vi "SpectrumAWG.vi"() -> ()   [LabVIEW 2014]
uses:
  Chart.ctl
  Wave.ctl
  spcm_library/spcm_gui_m4i.llb/element_ao_trigger.ctl
  spcm_library/spcm_gui_m4i.llb/element_clock.ctl
  spcm_library/spcm_gui_m4i.llb/element_ao_channel.ctl
  spcm_library/spcm_gui_m4i.llb/element_mode_out.ctl
panel:
  in  "Back":bool
  out "Wave Backup":T1 {"Phase (Pi)" min=-1.0 max=1.0 step=0.1 format="%.2f"; "Gap (us)" format="%.2f"; "Amplitude" format="%.2f"; "Duration (us)" format="%.2f"; "Frequency (MHz)" format="%.4f"}
  out "Card":cluster{"Card Handle":u64, "Error Code":u32}
  in  "Single":bool=TRUE
  in  "Formula":string="a*sin(w*t)" caption="data file"
  in  "Gap (us)":dbl=0.001 format="%.2f"
  in  "Phase (Pi)":dbl min=-1.0 max=1.0 step=0.1 format="%.2f"
  in  "Amplitude":dbl=1.0 format="%.2f"
  in  "Duration (us)":dbl=1.0 format="%.3f"
  in  "Frequency (MHz)":dbl=200.0 format="%.4f"
  in  "Output Channel":T2={"Enable"=TRUE, "Output Mode"=0, "Gain"=300, "Offset"=0, "Filter"=0} {"Output Mode" items=["Single", "Double", "Differential"]}
  in  "Mode":T3(ring)=enum."Single Restart"
  out "Status":string
  in  "Clock Settings":T4={"Clock Mode"=1, "Sampling Rate (MHz)"=1000.0, "Reference Clock (MHz)"=10.0, "Clock Output"=FALSE} {"Clock Mode" items=["Internal Clock Quartz", "External Clock (Reference Clock)", "Quartz 2 with PLL (Optional)"]; "Reference Clock (MHz)" min=10.0 max=125000.0; "Sampling Rate (MHz)" min=1.0 max=200000.0}
  in  "Trigger Settings":T5={"Trigger Source"=1, "Main Ext. Trigger"=2, "Level 0 Ext"=0, "Level 1 Ext"=0, "AC Coupling"=0, "Ext Trig Term"=FALSE, "Secondary Ext. Trigger"=0, "Level 0 Ext1"=0, "Trigger Delay (Samples)"=0} {"Secondary Ext. Trigger" items=["None", "Pos. Edge", "Neg. Edge", "Any Edge", "High Level", "Low Level"]; "AC Coupling" items=["DC Coupling", "AC Coupling"]; "Main Ext. Trigger" items=["None", "Pos. Edge", "Neg. Edge", "Any Edge", "Pos. Rearm", "Neg. Rearm", "Enter Window", "Leave Window", "High Level", "Low Level", "In Win", "Out Win", ""]; "Trigger Source" items=["Software Trigger", "Main External Trigger", "Secondary External Trigger"]; "Trigger Delay (Samples)" max=65535 step=1}
  in  "Sync":bool
  in  "Row":u16(ring) items=["0"]
  in  "Action":bool
  in  "Save":bool
  in  "SegmentPositions":i32[](array[numeric])
  in  "Wave File":path
  in  "Quit":bool
  in  "Steps":T6(array[cluster]) {"End" max=1 step=1}
  in  "Segment":u16(ring) items=["0"]
  out "Wave":T1 {"Phase (Pi)" min=-1.0 max=1.0 step=0.1 format="%.2f"; "Gap (us)" format="%.2f"; "Amplitude" format="%.2f"; "Duration (us)" format="%.3f"; "Frequency (MHz)" format="%.4f"}
  in  "Wave String":string="Frequency (MHz),Duration (us),Amplitude,Phase (Pi),Gap (us),Formula\n39,0,0.5,0,0,\n41,0,0.5,0,0,\n0,10,1,0,0,[0 1]"
  out "Plot":T7
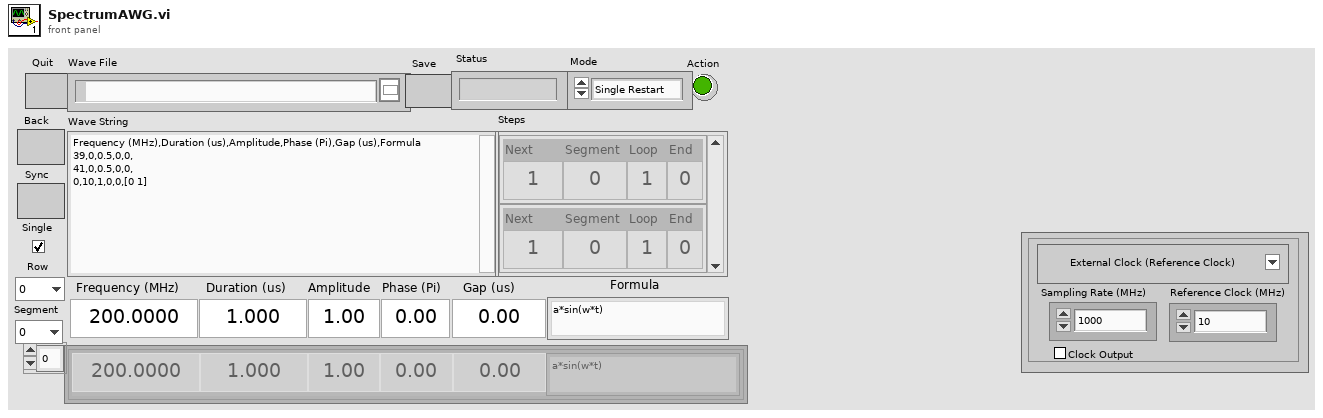
[diagram p1: front panel]
types:
  T1 = typedef "Wave.ctl" = cluster{"Frequency (MHz)":dbl, "Duration (us)":dbl, "Amplitude":dbl, "Phase (Pi)":dbl, "Gap (us)":dbl, "Formula":string}[]
  T2 = typedef "element_ao_channel.ctl" = cluster{"Enable":bool, "Output Mode":u16, "Gain":i32, "Offset":i32, "Filter":i32}
  T3 = enum16{"Singleshot", "Continuous", "Single Restart", "Multiple Replay", "Gated Replay"}
  T4 = typedef "element_clock.ctl" = cluster{"Clock Mode":u16, "Sampling Rate (MHz)":dbl, "Reference Clock (MHz)":dbl, "Clock Output":bool}
  T5 = typedef "element_ao_trigger.ctl" = cluster{"Trigger Source":u16, "Main Ext. Trigger":u16, "Level 0 Ext":i32, "Level 1 Ext":i32, "AC Coupling":u16, "Ext Trig Term":bool, "Secondary Ext. Trigger":u16, "Level 0 Ext1":i32, "Trigger Delay (Samples)":u32}
  T6 = cluster{"Next":u32, "Segment":u32, "Loop":u32, "End":u32}[]
  T7 = typedef "Chart.ctl" = waveform(dbl)
  T8 = cluster{"Index":u32, "IP Address":string, "Device":u16}
  T9 = cluster{"Next":u32, "Segment":u32, "Loop":u32, "End":u32}
  T10 = cluster{"Frequency (MHz)":dbl, "Duration (us)":dbl, "Amplitude":dbl, "Phase (Pi)":dbl, "Gap (us)":dbl, "Formula":string}
  T11 = typedef "element_mode_out.ctl" = cluster{"Mode":u16, "Mem":u32, "Seg":u32, "Loop":u32}
  T12 = cluster{"Number of segments":u32, "Start segment":u32}
  T13 = cluster{"Step":i32, "Next Step":i32, "Segment":i32, "Loops":i32, "End condition":u16}
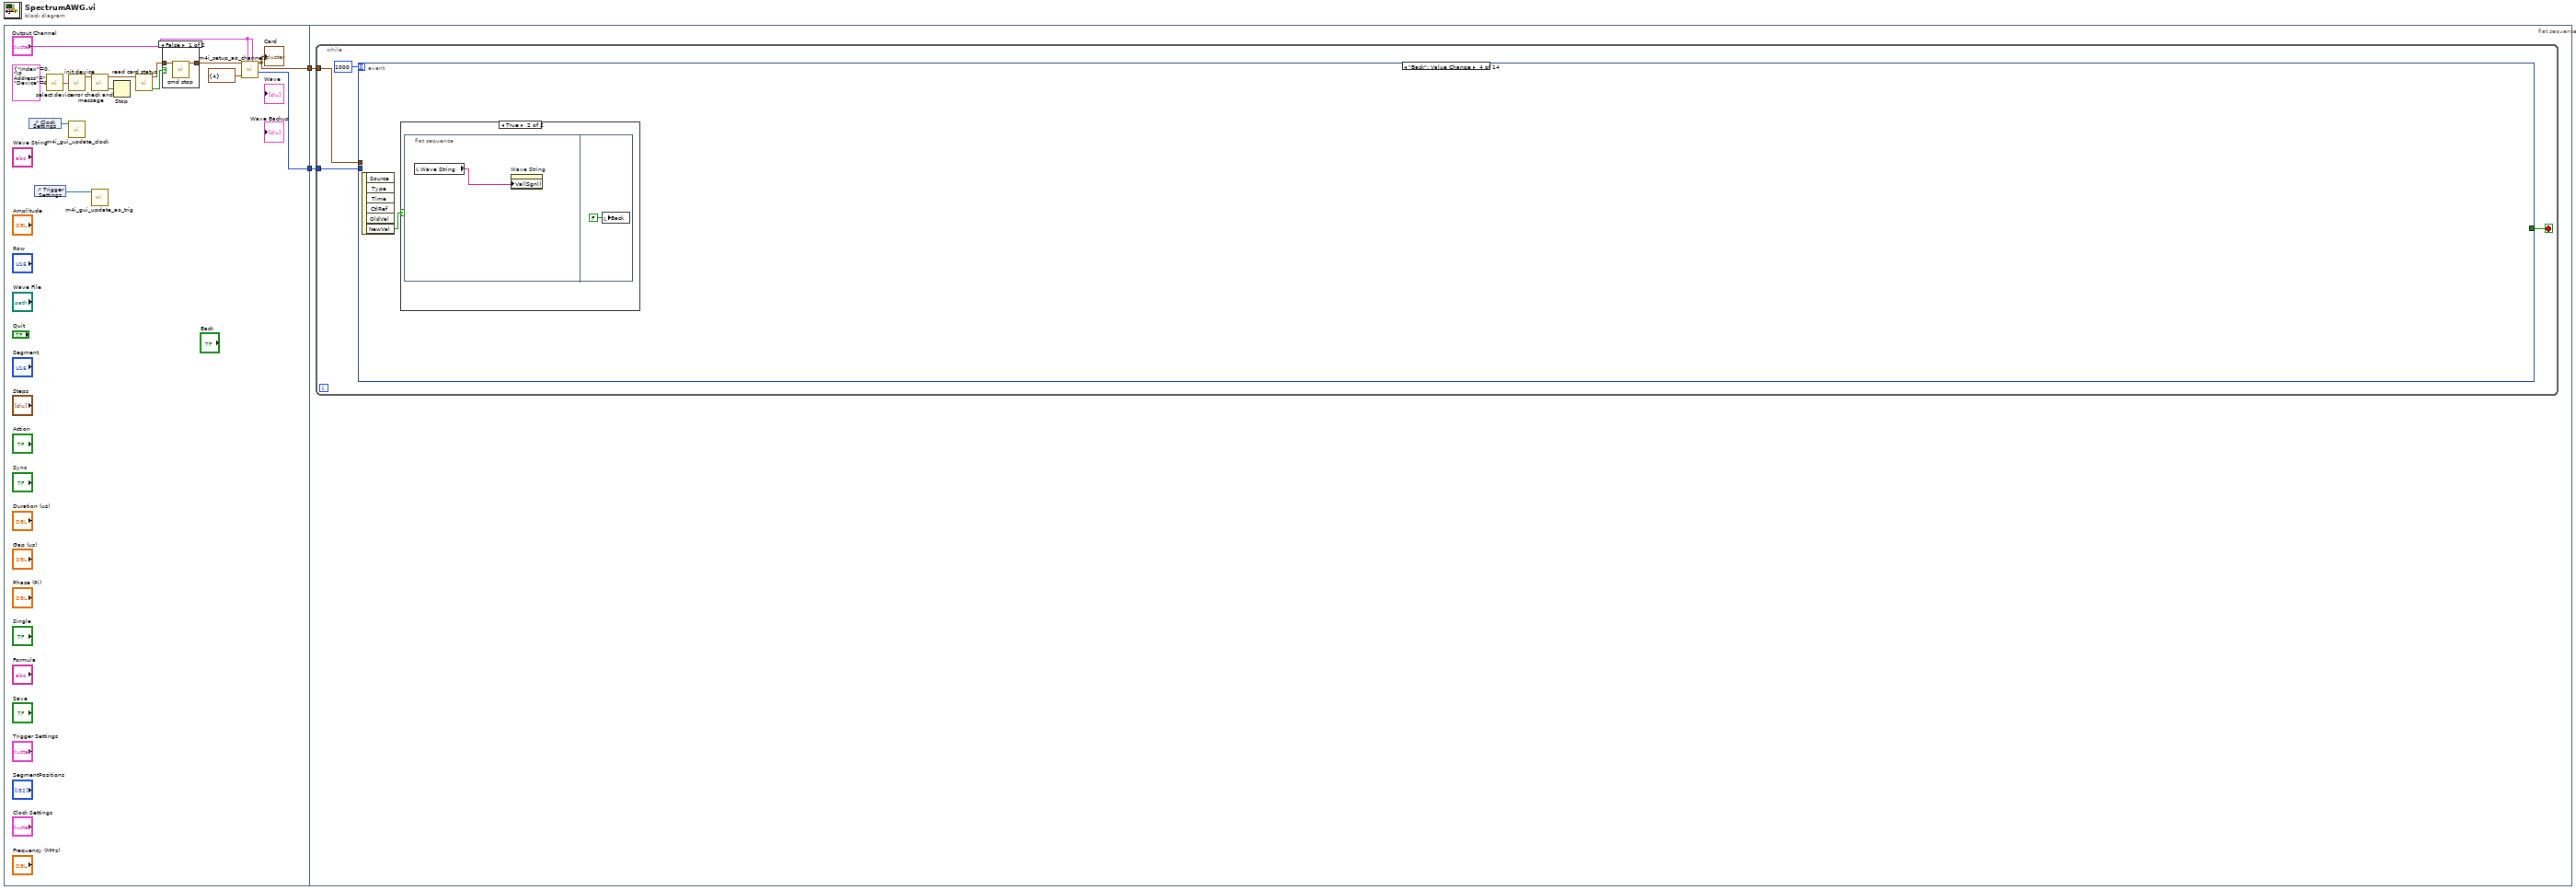
[diagram p0: block diagram]
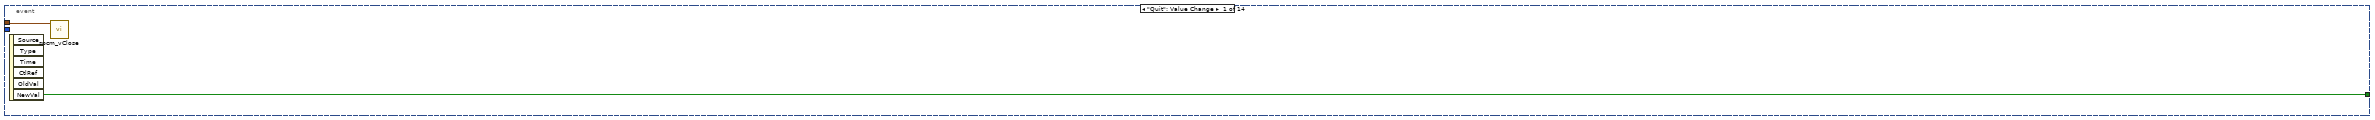
[diagram p3: hidden frame]
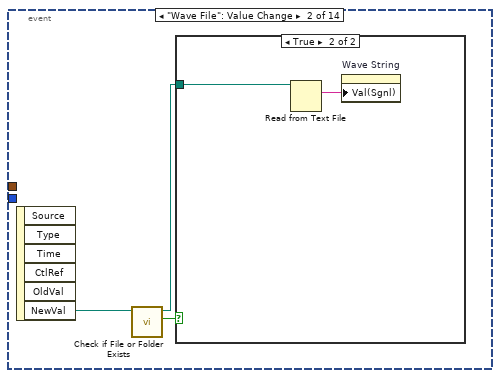
[diagram p4: hidden frame]
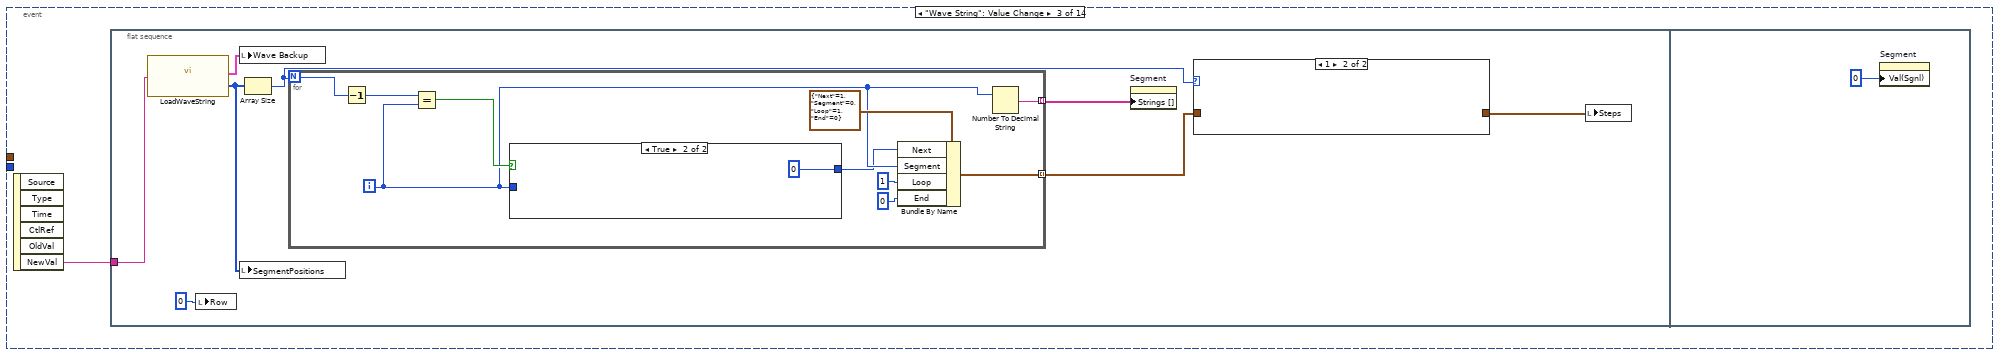
[diagram p6: hidden frame]
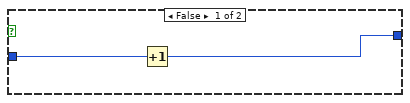
[diagram p8: hidden frame]
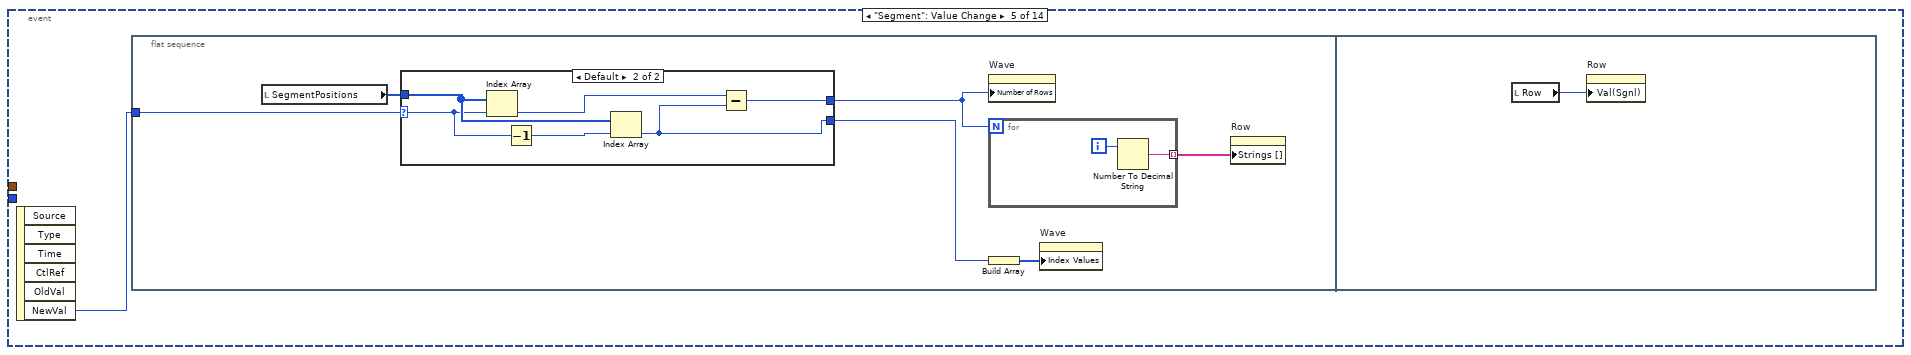
[diagram p10: hidden frame]
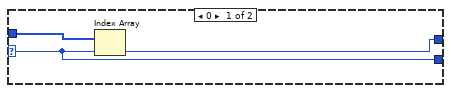
[diagram p11: hidden frame]
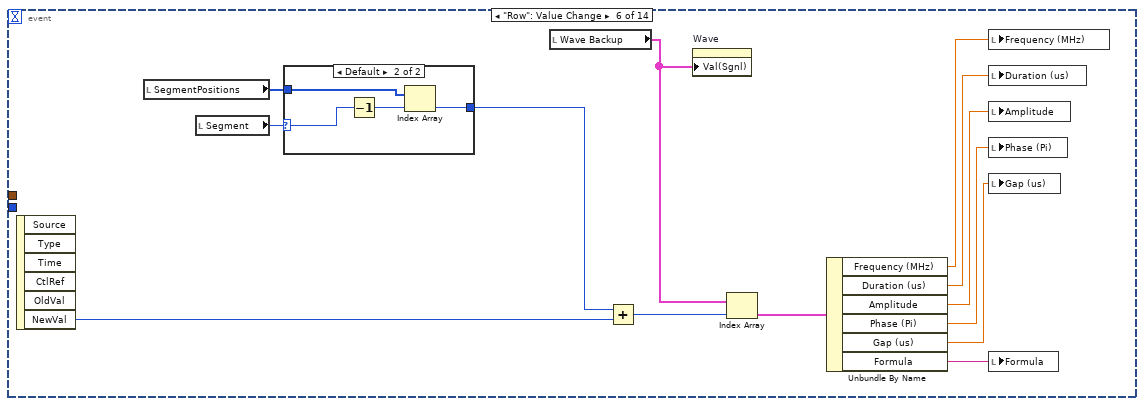
[diagram p12: hidden frame]
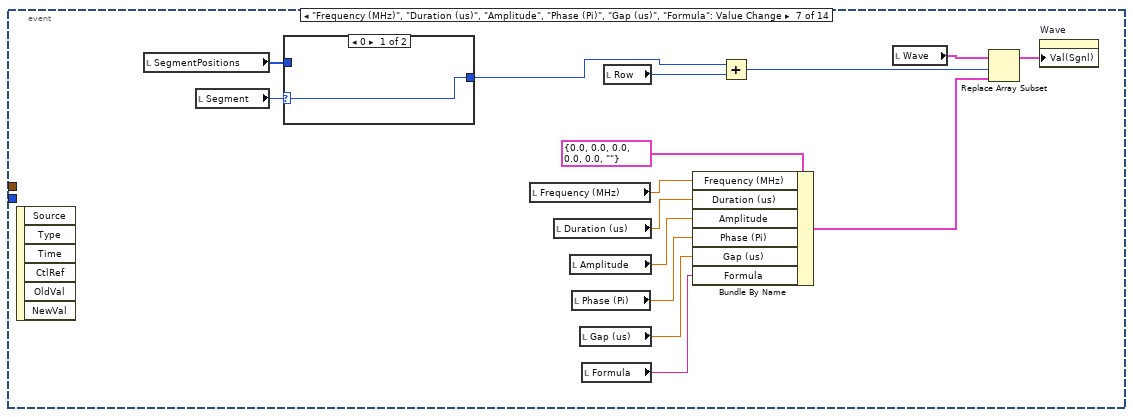
[diagram p14: hidden frame]
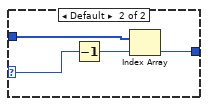
[diagram p15: hidden frame]
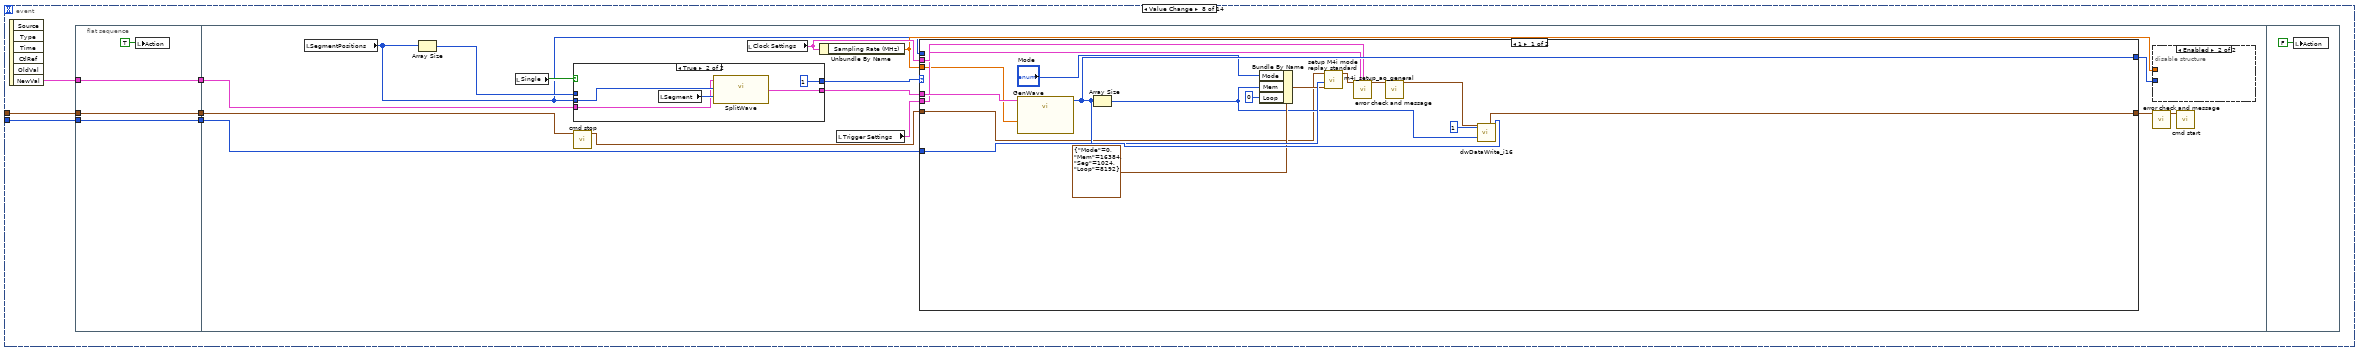
[diagram p16: hidden frame]
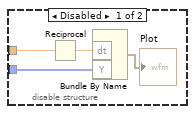
[diagram p18: hidden frame]
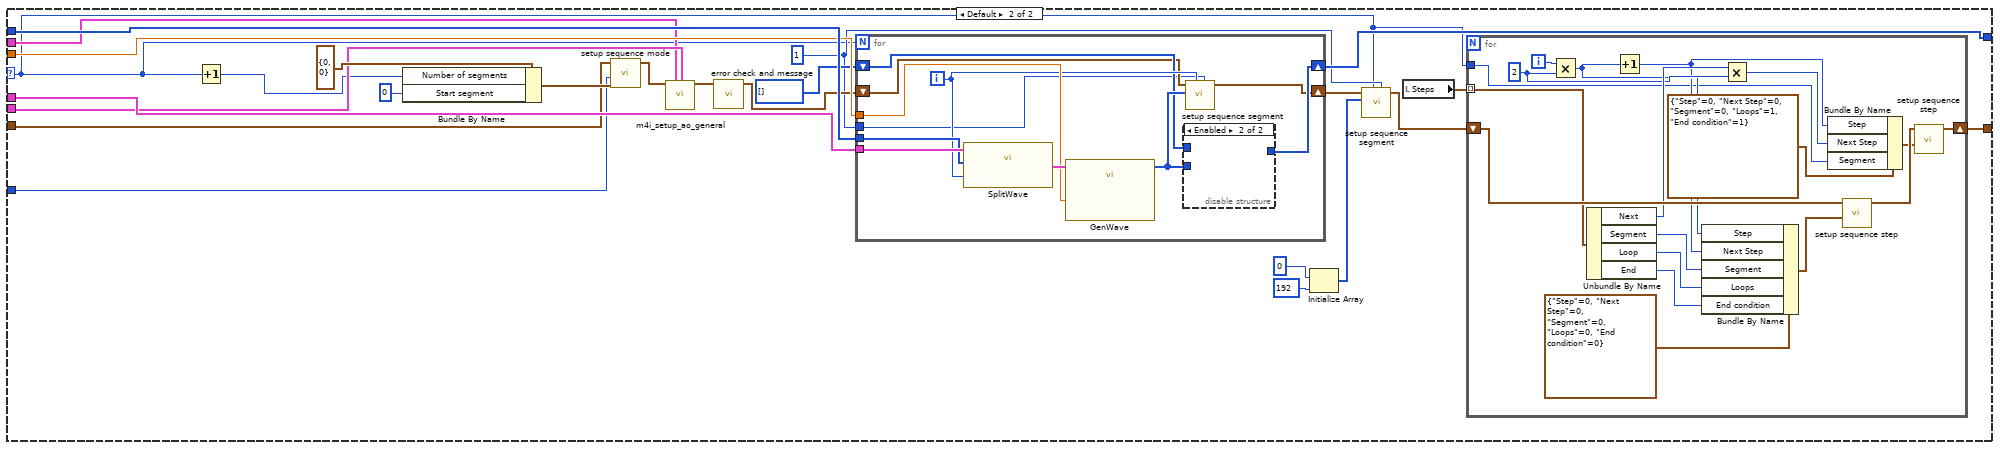
[diagram p19: hidden frame]
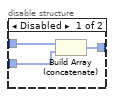
[diagram p20: hidden frame]
diagram:
  n1 = flat-sequence {
    tunnel: [w6] -> w2
    tunnel: [w3] -> w1
    tunnel: w2 -> [w21]
    tunnel: w1 -> [w20]
    frame #0 {
      n2 = control-ref of="Clock Settings"() -> (w7:refnum<vi>)
      n3 = control-ref of="Trigger Settings"() -> (w8:refnum<vi>)
      n4 = call "select device.vi"("Device"=T8 {"Index"=0, "IP Address"="", "Device"=0}) -> ("device string"=w16:string)  [unwired: 4 in]
      n5 = call "init device.vi"("Device String"=w16) -> ("Card Info Out"=w15:cluster{"Card Handle":u64, "Error Code":u32})  [unwired: 4 in, 1 out]
      n6 = call "m4i_gui_update_clock.vi"("Cluster Reference"=w7) -> ()  [unwired: 11 in]
      n7 = call "error check and message.vi"("Card Info In"=w15) -> ("Error occurred"=w14:bool, "Card Info Out"=w10:cluster{"Card Handle":u64, "Error Code":u32})  [unwired: 4 in, 1 out]
      n8 = call "m4i_gui_update_ao_trig.vi"("Cluster Referenz"=w8) -> ()  [unwired: 11 in]
      n9 = Stop(stop? (T)=w14) -> ()
      n10 = call "read card status.vi"("Card Info In"=w10) -> ("Card ready"=w11:bool, "Card Info Out"=w12:cluster{"Card Handle":u64, "Error Code":u32})  [unwired: 3 in, 2 out]
      n11 = case shown="False" w11 {
        tunnel: w12 -> [w18 w19]
        tunnel: [w17 w19] -> w9
        frame False {
          n12 = call "cmd stop.vi"("Card Info In"=w18) -> ("Card Info Out"=w17:cluster{"Card Handle":u64, "Error Code":u32})  [unwired: 6 in]
        }
        frame True {
        }
      }
      n13 = call "m4i_setup_ao_channels.vi"("Output Channel 1"="Output Channel", "Output Channel 0"="Output Channel", "Stop Level"=cluster{"Stoplevel":u16} {"Stoplevel"=4}, "Card Info In"=w9) -> ("ChMask"=w6:i32, "Card Info Out"=w3:cluster{"Card Handle":u64, "Error Code":u32})  [unwired: 5 in, 1 out]
      "Card" <- w3
    }
    frame #1 {
      n14 = while {
        tunnel: w21 -> [w24]
        tunnel: w20 -> [w22]
        stop <- w25 stop-if-true
        n15 = event shown="[3] \"Back\": Value Change" {
          selector: _ -> [_ _ _ _ _ _ _ _ _ _ _ _ _ _]
          dyn-events: _ -> [_ _ _ _ _ _ _ _ _ _ _ _ _ _]
          timeout: 1000 -> [_ _ _ _ _ _ _ _ _ _ _ _ _ _]
          tunnel: [w27 _ _ _ _ _ _ _ _ _ _ _ _ _] -> w25
          tunnel: w22 -> [w26 _ _ _ _ _ _ w121 _ _ _ w271 w301 _]
          tunnel: w24 -> [_ _ _ _ _ _ _ w120 _ _ _ _ _ _]
          event "Quit": Value Change {
            n16 = event-data() -> ("NewVal"=w27:bool)  [unwired: 1 in, 5 out]
            n17 = call "spcm_vClose.vi"("Card Info In"=w26) -> ()  [unwired: 7 in]
          }
          event "Wave File": Value Change {
            n18 = event-data() -> ("NewVal"=w30:path)  [unwired: 1 in, 5 out]
            n19 = call <vilib>:"Check if File or Folder Exists.vi"("path"=w30) -> ("file or folder exists?"=w29:bool, "dup path"=w28:path)  [unwired: 8 in, 1 out]
            n20 = case shown="True" w29 {
              tunnel: w28 -> [_ w31]
              frame False {
              }
              frame True {
                n21 = Read from Text File(file (use dialog)=w31) -> (text=w32:string)  [unwired: 3 in, 3 out]
                n22 = property on="Wave String" class="Str"("Val(Sgnl)"=w32) -> ()  [unwired: 2 in, 2 out]
              }
            }
          }
          event "Wave String": Value Change {
            n23 = event-data() -> ("NewVal"=w33:string)  [unwired: 1 in, 5 out]
            n24 = flat-sequence {
              tunnel: w33 -> [w41]
              frame #0 {
                n25 = call "LoadWaveString.vi"("Wave String"=w41) -> ("All Wave"=w34:T1, "SegmentPositions"=w37:i32[])  [unwired: 1 out]
                n26 = local write "Row"(0) -> ()
                n27 = local write "Wave Backup"(w34) -> ()
                n28 = local write "SegmentPositions"(w37) -> ()
                n29 = Array Size(array=w37) -> (size(s)=w36:i32)
                n30 = for {
                  N: w36 -> [w49]
                  tunnel: [w52] -> w40 mode=indexing
                  tunnel: [w46] -> w39 mode=indexing
                  i -> [w44]
                  n31 = Decrement(x=w49) -> (x-1=w48:i32)
                  n32 = Equal?(x=w48, y=w44) -> (x = y?=w47:bool)
                  n33 = case shown="True" w47 {
                    tunnel: [w53 u32 0 ("End")] -> w43
                    tunnel: w44 -> [w54 _]
                    frame False {
                      n34 = Increment(x=w54) -> (x+1=w53:i32)
                    }
                    frame True {
                    }
                  }
                  n35 = Bundle By Name(cluster=T9 {"Next"=1, "Segment"=0, "Loop"=1, "End"=0} ("input cluster 2"), "Next"=w43, "Segment"=w44, "Loop"=u32 1, "End"=u32 0) -> (w46:T9)
                  n36 = Number To Decimal String(number=w44) -> (decimal integer string=w52:string)  [unwired: 1 in]
                }
                n37 = property on="Segment" class="Ring (strict)"("Strings []"=w40) -> ()  [unwired: 2 in, 2 out]
                n38 = case shown="1" w36 {
                  tunnel: w39 -> [w42 _]
                  tunnel: [w42 _] -> w38
                  frame Default {
                  }
                  frame 1 {
                  }
                }
                n39 = local write "Steps"(w38) -> ()
              }
              frame #1 {
                n40 = property on="Segment" class="Ring (strict)"("Val(Sgnl)"=u16 0 ("Value (Signaling)")) -> ()  [unwired: 2 in, 2 out]
              }
            }
          }
          event "Back": Value Change {
            n41 = event-data() -> ("NewVal"=w57:bool)  [unwired: 1 in, 5 out]
            n42 = case shown="True" w57 {
              frame False {
              }
              frame True {
                n43 = flat-sequence {
                  frame #0 {
                    n44 = local read "Wave String"() -> (w58:string)
                    n45 = property on="Wave String" class="Str"("Val(Sgnl)"=w58) -> ()  [unwired: 2 in, 2 out]
                  }
                  frame #1 {
                    n46 = local write "Back"(FALSE ("Back")) -> ()
                  }
                }
              }
            }
          }
          event "Segment": Value Change {
            n47 = event-data() -> ("NewVal"=w60:u16)  [unwired: 1 in, 5 out]
            n48 = flat-sequence {
              tunnel: w60 -> [w66]
              frame #0 {
                n49 = local read "SegmentPositions"() -> (w63:i32[])
                n50 = case shown="Default" w66 {
                  selector: w66 -> [w71 w75]
                  tunnel: [w71 w73] -> w65
                  tunnel: w63 -> [w70 w76]
                  tunnel: [w69 w72] -> w62
                  frame 0 {
                    n51 = Index Array(array=w70, index=w71) -> (element=w69:i32)
                  }
                  frame Default {
                    n52 = Index Array(array=w76, index=w75) -> (element=w74:i32)
                    n53 = Decrement(x=w75) -> (x-1=w77:u16)
                    n54 = Index Array(array=w76, index=w77) -> (element=w73:i32)
                    n55 = Subtract(x=w74, y=w73) -> (x-y=w72:i32)
                  }
                }
                n56 = property on="Wave" class="Arr (strict)"("Number of Rows"=w62) -> ()  [unwired: 2 in, 2 out]
                n57 = for {
                  N: w62 -> [_]
                  tunnel: [w67] -> w61 mode=indexing
                  i -> [w68]
                  n58 = Number To Decimal String(number=w68) -> (decimal integer string=w67:string)  [unwired: 1 in]
                }
                n59 = Build Array(w65) -> (w64:i32[])
                n60 = property on="Wave" class="Arr (strict)"("Index Values"=w64) -> ()  [unwired: 2 in, 2 out]
                n61 = property on="Row" class="Ring (strict)"("Strings []"=w61) -> ()  [unwired: 2 in, 2 out]
              }
              frame #1 {
                n62 = local read "Row"() -> (w78:u16)
                n63 = property on="Row" class="Ring (strict)"("Val(Sgnl)"=w78) -> ()  [unwired: 2 in, 2 out]
              }
            }
          }
          event "Row": Value Change {
            n64 = event-data() -> ("NewVal"=w89:u16)  [unwired: 1 in, 5 out]
            n65 = local read "SegmentPositions"() -> (w91:i32[])
            n66 = local read "Segment"() -> (w88:u16)
            n67 = case shown="Default" w88 {
              selector: w88 -> [w92 w94]
              tunnel: [w92 w93] -> w90
              tunnel: w91 -> [_ w95]
              frame 0 {
              }
              frame Default {
                n68 = Decrement(x=w94) -> (x-1=w96:u16)
                n69 = Index Array(array=w95, index=w96) -> (element=w93:i32)
              }
            }
            n70 = local read "Wave Backup"() -> (w79:T1)
            n71 = Add(x=w90, y=w89) -> (x+y=w87:i32)
            n72 = property on="Wave" class="Arr (strict)"("Val(Sgnl)"=w79) -> ()  [unwired: 2 in, 2 out]
            n73 = Index Array(array=w79, index=w87) -> (element=w86:T10)
            n74 = Unbundle By Name(w86) -> ("Frequency (MHz)"=w85:dbl, "Duration (us)"=w84:dbl, "Amplitude"=w83:dbl, "Phase (Pi)"=w82:dbl, "Gap (us)"=w81:dbl, "Formula"=w80:string)
            n75 = local write "Frequency (MHz)"(w85) -> ()
            n76 = local write "Duration (us)"(w84) -> ()
            n77 = local write "Amplitude"(w83) -> ()
            n78 = local write "Phase (Pi)"(w82) -> ()
            n79 = local write "Gap (us)"(w81) -> ()
            n80 = local write "Formula"(w80) -> ()
          }
          event "Frequency (MHz)", "Duration (us)", "Amplitude", "Phase (Pi)", "Gap (us)", "Formula": Value Change {
            n81 = event-data() -> ()  [unwired: 1 in, 6 out]
            n82 = local read "SegmentPositions"() -> (w111:i32[])
            n83 = local read "Segment"() -> (w109:u16)
            n84 = case shown="0" w109 {
              selector: w109 -> [w112 w114]
              tunnel: [w112 w113] -> w110
              tunnel: w111 -> [_ w115]
              frame 0 {
              }
              frame Default {
                n85 = Decrement(x=w114) -> (x-1=w116:u16)
                n86 = Index Array(array=w115, index=w116) -> (element=w113:i32)
              }
            }
            n87 = local read "Frequency (MHz)"() -> (w103:dbl)
            n88 = local read "Duration (us)"() -> (w102:dbl)
            n89 = local read "Amplitude"() -> (w101:dbl)
            n90 = local read "Phase (Pi)"() -> (w100:dbl)
            n91 = local read "Gap (us)"() -> (w99:dbl)
            n92 = local read "Formula"() -> (w98:string)
            n93 = local read "Row"() -> (w108:u16)
            n94 = Bundle By Name(cluster=T10 {"Frequency (MHz)"=0.0, "Duration (us)"=0.0, "Amplitude"=0.0, "Phase (Pi)"=0.0, "Gap (us)"=0.0, "Formula"=""} ("Wave"), "Frequency (MHz)"=w103, "Duration (us)"=w102, "Amplitude"=w101, "Phase (Pi)"=w100, "Gap (us)"=w99, "Formula"=w98) -> (w97:T10)
            n95 = Add(x=w110, y=w108) -> (x+y=w106:i32)
            n96 = local read "Wave"() -> (w107:T1)
            n97 = Replace Array Subset(array=w107, new element=w97, index=w106) -> (w105:T1)
            n98 = property on="Wave" class="Arr (strict)"("Val(Sgnl)"=w105) -> ()  [unwired: 2 in, 2 out]
          }
          event Value Change {
            n99 = event-data() -> ("NewVal"=w122:T1)  [unwired: 1 in, 5 out]
            n100 = flat-sequence {
              tunnel: w120 -> [w124]
              tunnel: w121 -> [w125]
              tunnel: w122 -> [w126]
              tunnel: [w126] -> w119
              tunnel: [w125] -> w118
              tunnel: [w124] -> w117
              tunnel: w119 -> [w131]
              tunnel: w118 -> [w128]
              tunnel: w117 -> [w140]
              frame #0 {
                n101 = local write "Action"(TRUE ("Busy")) -> ()
              }
              frame #1 {
                n102 = local read "SegmentPositions"() -> (w129:i32[])
                n103 = Array Size(array=w129) -> (size(s)=w133:i32)
                n104 = local read "Single"() -> (w134:bool)
                n105 = case shown="True" w134 {
                  tunnel: w133 -> [w143 _]
                  tunnel: [w143 1] -> w132
                  tunnel: w131 -> [w142 w145]
                  tunnel: [w142 w144] -> w130
                  tunnel: w129 -> [_ w146]
                  frame False {
                  }
                  frame True {
                    n106 = local read "Segment"() -> (w147:u16)
                    n107 = call "SplitWave.vi"("Index"=w147, "SegmentPositions"=w146, "All Wave"=w145) -> ("Wave"=w144:T1)
                  }
                }
                n108 = call "cmd stop.vi"("Card Info In"=w128) -> ("Card Info Out"=w127:cluster{"Card Handle":u64, "Error Code":u32})  [unwired: 6 in]
                n109 = local read "Clock Settings"() -> (w139:T4)
                n110 = Unbundle By Name(w139) -> ("Sampling Rate (MHz)"=w137:dbl)
                n111 = local read "Trigger Settings"() -> (w138:T5)
                n112 = case shown="1" w132 {
                  selector: w132 -> [_ w173]
                  tunnel: w130 -> [w169 w191]
                  tunnel: w129 -> [_ w190]
                  tunnel: w127 -> [w153 w170]
                  tunnel: [w168 w187] -> w141
                  tunnel: w140 -> [w167 w171]
                  tunnel: [w166 w185] -> w136
                  tunnel: w139 -> [w165 w180]
                  tunnel: w138 -> [w164 w181]
                  tunnel: w137 -> [w163 w189]
                  frame 1 {
                    n113 = call "GenWave.vi"("Sampling Rate (MHz)"=w163, "Wave"=w169) -> ("Output"=w168:i16[])  [unwired: 4 in, 1 out]
                    n114 = Array Size(array=w168) -> (size(s)=w158:i32)
                    n115 = Bundle By Name(cluster=T11 {"Mode"=0, "Mem"=16384, "Seg"=1024, "Loop"=8192} ("Mode Out Setup"), "Mode"="Mode", "Mem"=w158, "Loop"=u32 0) -> (w159:T11)
                    n116 = call "setup M4i mode replay standard.vi"("Mode Out Setup"=w159, "Channel Mask Low"=w167, "Card Info In"=w153) -> ("Card Info Out"=w156:cluster{"Card Handle":u64, "Error Code":u32})  [unwired: 4 in]
                    n117 = call "m4i_setup_ao_general.vi"("Card Info In"=w156, "Clock Settings"=w165, "Trigger Settings"=w164) -> ("Card Info Out"=w155:cluster{"Card Handle":u64, "Error Code":u32})  [unwired: 8 in, 4 out]
                    n118 = call "error check and message.vi"("Card Info In"=w155) -> ("Card Info Out"=w154:cluster{"Card Handle":u64, "Error Code":u32})  [unwired: 4 in, 2 out]
                    n119 = call "dwDataWrite_i16.vi"("Card Info In"=w154, "Channel Count"=u32 1, "Length (Samples per Channel)"=w158, "Ch 0"=w168) -> ("Card Info Out"=w166:cluster{"Card Handle":u64, "Error Code":u32})  [unwired: 23 in]
                  }
                  frame Default {
                    w177 = 1 ("Number of channels")
                    n120 = Increment(x=w173) -> (x+1=w172:i32)
                    n121 = Bundle By Name(cluster=T12 {"Number of segments"=0, "Start segment"=0} ("Sequence Mode Setup"), "Number of segments"=w172, "Start segment"=u32 0) -> (w192:T12)
                    n122 = call "setup sequence mode.vi"("Sequence Mode Setup"=w192, "Channel  Mask Low"=w171, "Card Info In"=w170) -> ("Card Info Out"=w183:cluster{"Card Handle":u64, "Error Code":u32})  [unwired: 8 in]
                    n123 = call "m4i_setup_ao_general.vi"("Card Info In"=w183, "Clock Settings"=w180, "Trigger Settings"=w181) -> ("Card Info Out"=w184:cluster{"Card Handle":u64, "Error Code":u32})  [unwired: 8 in, 4 out]
                    n124 = call "error check and message.vi"("Card Info In"=w184) -> ("Card Info Out"=w182:cluster{"Card Handle":u64, "Error Code":u32})  [unwired: 4 in, 2 out]
                    n125 = for {
                      N: w173 -> [_]
                      tunnel: w191 -> [w223]
                      tunnel: w190 -> [w222]
                      tunnel: w189 -> [w220]
                      shift-right: [w217] -> w187
                      shift-left: i16[] [] ("Output") -> [w216]
                      shift-right: [w215] -> w179
                      shift-left: w182 -> [w214]
                      tunnel: w177 -> [w213]
                      i -> [w219]
                      n126 = call "SplitWave.vi"("Index"=w219, "SegmentPositions"=w222, "All Wave"=w223) -> ("Wave"=w221:T1)
                      n127 = call "GenWave.vi"("Sampling Rate (MHz)"=w220, "Wave"=w221) -> ("Output"=w218:i16[])  [unwired: 4 in, 1 out]
                      n128 = disable-structure shown="Enabled" {
                        disable-tunnel: w218 -> [w226 _]
                        disable-tunnel: [w225 _] -> w217
                        disable-tunnel: w216 -> [w224 _]
                        frame Disabled {
                          n129 = Build Array (concatenate)(w224, w226) -> (w225:i16[])
                        }
                        frame Enabled {
                        }
                      }
                      n130 = call "setup sequence segment.vi"("Number of channels"=w213, "Segment number"=w219, "Segment Data Ch0"=w218, "Card Info In"=w214) -> ("Card Info Out"=w215:cluster{"Card Handle":u64, "Error Code":u32})  [unwired: 7 in]
                    }
                    n131 = Initialize Array(i16 0, 192 ("dimension size")) -> (w174:i16[])
                    n132 = call "setup sequence segment.vi"("Number of channels"=w177, "Segment number"=w173, "Segment Data Ch0"=w174, "Card Info In"=w179) -> ("Card Info Out"=w178:cluster{"Card Handle":u64, "Error Code":u32})  [unwired: 7 in]
                    n133 = local read "Steps"() -> (w186:T6)
                    n134 = for {
                      shift-right: [w204] -> w185
                      shift-left: w178 -> [w208]
                      tunnel: w186 -> [w207] mode=indexing
                      tunnel: w173 -> [w195]
                      i -> [w201]
                      w199 = 2 ("Loops")
                      n135 = Multiply(x=w201, y=w199) -> (x*y=w198:i32)
                      n136 = Unbundle By Name(w207) -> ("Next"=w200:u32, "Segment"=w210:u32, "Loop"=w211:u32, "End"=w212:u32)
                      n137 = Increment(x=w198) -> (x+1=w196:i32)
                      n138 = Bundle By Name(cluster=T13 {"Step"=0, "Next Step"=0, "Segment"=0, "Loops"=0, "End condition"=0} ("Sequence Step"), "Step"=w198, "Next Step"=w196, "Segment"=w210, "Loops"=w211, "End condition"=w212) -> (w206:T13)
                      n139 = Multiply(x=w200, y=w199) -> (x*y=w197:u32)
                      n140 = Bundle By Name(cluster=T13 {"Step"=0, "Next Step"=0, "Segment"=0, "Loops"=1, "End condition"=1} ("Sequence Step"), "Step"=w196, "Next Step"=w197, "Segment"=w195) -> (w202:T13)
                      n141 = call "setup sequence step.vi"("Sequence Step"=w206, "Card Info In"=w208) -> ("Card Info Out"=w205:cluster{"Card Handle":u64, "Error Code":u32})  [unwired: 9 in]
                      n142 = call "setup sequence step.vi"("Sequence Step"=w202, "Card Info In"=w205) -> ("Card Info Out"=w204:cluster{"Card Handle":u64, "Error Code":u32})  [unwired: 9 in]
                    }
                  }
                }
                n143 = disable-structure shown="Enabled" {
                  disable-tunnel: w141 -> [w150 _]
                  disable-tunnel: w137 -> [w149 _]
                  frame Disabled {
                    n144 = Reciprocal(x=w149) -> (1/x=w151:dbl)
                    n145 = Bundle By Name("dt"=w151, "Y"=w150) -> (→"Plot":waveform(i16))  [unwired: 1 in]
                  }
                  frame Enabled {
                  }
                }
                n146 = call "error check and message.vi"("Card Info In"=w136) -> ("Card Info Out"=w135:cluster{"Card Handle":u64, "Error Code":u32})  [unwired: 4 in, 2 out]
                n147 = call "cmd start.vi"("Card Info In"=w135) -> ()  [unwired: 6 in, 1 out]
              }
              frame #2 {
                n148 = local write "Action"(FALSE ("Busy")) -> ()
              }
            }
          }
          event Value Change {
            n149 = event-data() -> ()  [unwired: 1 in, 6 out]
            n150 = control-ref of="Clock Settings"() -> (w228:refnum<vi>)
            n151 = call "m4i_gui_update_clock.vi"("Cluster Reference"=w228) -> ()  [unwired: 11 in]
          }
          event Value Change {
            n152 = event-data() -> ()  [unwired: 1 in, 6 out]
            n153 = control-ref of="Trigger Settings"() -> (w229:refnum<vi>)
            n154 = call "m4i_gui_update_ao_trig.vi"("Cluster Referenz"=w229) -> ()  [unwired: 11 in]
          }
          event "Sync": Value Change {
            n155 = event-data() -> ("NewVal"=w230:bool)  [unwired: 1 in, 5 out]
            n156 = case shown="True" w230 {
              frame False {
              }
              frame True {
                n157 = flat-sequence {
                  frame #0 {
                    n158 = local read "SegmentPositions"() -> (w232:i32[])
                    n159 = local read "Wave"() -> (w235:T1)
                    n160 = for {
                      tunnel: w235 -> [w262] mode=indexing
                      shift-right: [w240] -> w233
                      shift-left: "Frequency (MHz),Duration (us),Amplitude,Phase (Pi),Gap (us),Formula\n" -> [w246]
                      tunnel: w232 -> [w245]
                      shift-right: [w236] -> _
                      shift-left: i16 0 ("precision (6)") -> [w237]
                      i -> [w239]
                      w241 = "\r\n"
                      w254 = i16 2 ("precision (6)")
                      w248 = "," ("string")
                      n161 = Unbundle By Name(w262) -> ("Frequency (MHz)"=w261:dbl, "Duration (us)"=w257:dbl, "Amplitude"=w256:dbl, "Phase (Pi)"=w255:dbl, "Gap (us)"=w253:dbl, "Formula"=w247:string)
                      n162 = Index Array(array=w245, index=w237) -> (element=w244:i32)
                      n163 = Number To Fractional String(number=w256, precision (6)=w254) -> (F-format string=w251:string)  [unwired: 2 in]
                      n164 = Number To Fractional String(number=w255, precision (6)=w254) -> (F-format string=w250:string)  [unwired: 2 in]
                      n165 = Number To Fractional String(number=w253, precision (6)=w254) -> (F-format string=w249:string)  [unwired: 2 in]
                      n166 = Number To Fractional String(number=w261, precision (6)=i16 4) -> (F-format string=w259:string)  [unwired: 2 in]
                      n167 = Number To Fractional String(number=w257, precision (6)=i16 3) -> (F-format string=w252:string)  [unwired: 2 in]
                      n168 = Increment(x=w239) -> (x+1=w238:i32)
                      n169 = Equal?(x=w244, y=w238) -> (x = y?=w243:bool)
                      n170 = Concatenate Strings(w246, w259, w248, w252, w248, w251, w248, w250, w248, w249, w248, w247, w241) -> (w242:string)
                      n171 = case shown="False" w243 {
                        tunnel: w242 -> [w263 w269]
                        tunnel: w241 -> [_ w268]
                        tunnel: [w263 w267] -> w240
                        tunnel: w237 -> [w264 w266]
                        tunnel: [w264 w265] -> w236
                        frame False {
                        }
                        frame True {
                          n172 = Increment(x=w266) -> (x+1=w265:i16)
                          n173 = Concatenate Strings(w269, w268) -> (w267:string)
                        }
                      }
                    }
                    n174 = local write "Wave String"(w233) -> ()
                  }
                  frame #1 {
                    n175 = local write "Sync"(FALSE ("Reload")) -> ()
                  }
                }
              }
            }
          }
          event "Action": Value Change {
            n176 = event-data() -> ("NewVal"=w272:bool)  [unwired: 1 in, 5 out]
            n177 = case shown="True" w272 {
              tunnel: w271 -> [_ w281]
              frame False {
              }
              frame True {
                n178 = flat-sequence {
                  tunnel: w281 -> [w288]
                  tunnel: [w285] -> w279
                  tunnel: [w284] -> w277
                  tunnel: [w283] -> w275
                  tunnel: [w282] -> w274
                  tunnel: [w289] -> w280
                  tunnel: w279 -> [w290]
                  tunnel: [w293] -> w278
                  tunnel: w277 -> [w293]
                  tunnel: [w292] -> w276
                  tunnel: w275 -> [w292]
                  tunnel: w274 -> [w291]
                  tunnel: [w291] -> w273
                  tunnel: w280 -> [w298]
                  tunnel: w278 -> [w297]
                  tunnel: w276 -> [w296]
                  tunnel: w273 -> [w295]
                  frame #0 {
                    w287 = u16 0 items=["Software Trigger", "Main External Trigger", "Secondary External Trigger"] ("Trigger Source")
                    n179 = local read "Trigger Settings"() -> (w283:T5)
                    n180 = Bundle By Name(cluster=w283, "Trigger Source"=w287) -> (w286:T5)
                    n181 = Unbundle By Name(w283) -> ("Trigger Source"=w282:u16)
                    n182 = local read "Clock Settings"() -> (w284:T4)
                    n183 = call "m4i_setup_ao_general.vi"("Card Info In"=w288, "Clock Settings"=w284, "Trigger Settings"=w286) -> ("Card Info Out"=w285:cluster{"Card Handle":u64, "Error Code":u32})  [unwired: 8 in, 4 out]
                  }
                  frame #1 {
                    n184 = call "cmd force trigger.vi"("Card Info In"=w290) -> ("Card Info Out"=w289:cluster{"Card Handle":u64, "Error Code":u32})  [unwired: 6 in]
                  }
                  frame #2 {
                    n185 = Bundle By Name(cluster=w296, "Trigger Source"=w295) -> (w294:T5)
                    n186 = call "m4i_setup_ao_general.vi"("Card Info In"=w298, "Clock Settings"=w297, "Trigger Settings"=w294) -> ()  [unwired: 8 in, 5 out]
                  }
                  frame #3 {
                    n187 = local write "Action"(FALSE ("Data")) -> ()
                  }
                }
              }
            }
          }
          event Timeout {
            n188 = event-data() -> ()  [unwired: 1 in, 3 out]
            n189 = call "read card status.vi"("Card Info In"=w301) -> ("Card ready"=w303:bool, "Trigger detected"=w304:bool, "Pretrigger full"=w305:bool, "Card Info Out"=w302:cluster{"Card Handle":u64, "Error Code":u32})  [unwired: 3 in]
            n190 = call "error check and message.vi"("Card Info In"=w302) -> ()  [unwired: 4 in, 3 out]
            n191 = call "spcm_translate_status_out.vi"("Ready"=w303, "Trigger"=w304, "Pretrigger"=w305) -> ("Text"=→"Status":string)  [unwired: 4 in]
          }
          event "Save": Value Change {
            n192 = event-data() -> ("NewVal"=w306:bool)  [unwired: 1 in, 5 out]
            n193 = case shown="True" w306 {
              frame False {
              }
              frame True {
                n194 = flat-sequence {
                  frame #0 {
                    n195 = local read "Wave String"() -> (w308:string)
                    n196 = local read "Wave File"() -> (w307:path)
                    n197 = Write to Text File(file (use dialog)=w307, text=w308) -> ()  [unwired: 2 in, 3 out]
                  }
                  frame #1 {
                    n198 = local write "Save"(FALSE ("Save")) -> ()
                  }
                }
              }
            }
          }
        }
      }
    }
  }
